vi "i_Gyro.vi"(3 "LocalDataOut":cluster{}, 11 "LocalDataIn":cluster{}) -> ()   [LabVIEW 2017]
uses:
  <vilib>/Rock Robotics/Network Tables/NT Write Number.vi
panel:
  in  "RefnumName":string
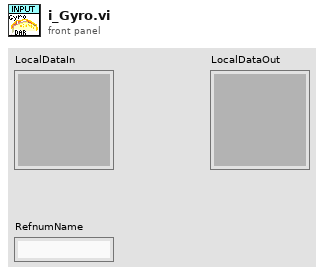
[diagram p1: front panel]
types:
  T1 = typedef "WPI_GyroDevRef.ctl" = cluster{"DevStatus":errorcluster, "Analog Channel":T2, "Gain (VoltsPerDegree/Second)":dbl, "Gyro Type":enum16{"Analog", "XRS450"}, "Handle":i32, "SPI Bus":T3, "Device Found":bool, "Sample Rate":dbl, "Calibrate On Open":bool, "Offset":dbl}
  T2 = typedef "FPGA_AIChannel.ctl" = enum8{"AI 0", "AI 1", "AI 2", "AI 3", "AI MXP 0", "AI MXP 1", "AI MXP 2", "AI MXP 3", "Invalid"}
  T3 = typedef "spi_bus.ctl" = enum16{"SPI On-Board, CS0", "SPI On-Board, CS1", "SPI On-Board, CS2", "SPI On-Board, CS3", "SPI MXP", "Invalid"}
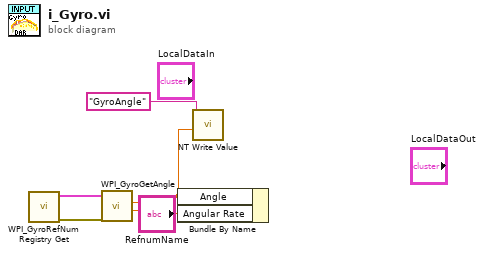
[diagram p0: block diagram]
diagram:
  n1 = call <vilib>:"WPI_GyroRefNum Registry Get.vi"() -> ("error out"=w2:errorcluster, "GyroDevRef"=w5:T1)  [unwired: 10 in]
  n2 = call <vilib>:"WPI_GyroGetAngle.vi"("error in (no error)"=w2, "GyroDevRef"=w5) -> ("Angular Rate"=w4:dbl, "Angle"=w3:dbl)  [unwired: 6 in, 2 out]
  n3 = Bundle By Name("Angle"=w3, "Angular Rate"=w4) -> ()  [unwired: 1 in, 1 out]
  n4 = call-poly <vilib>:"NT Write Value.vi"("Numeric"=w3, "Name"="GyroAngle") -> ()  [unwired: 9 in, 1 out]
